vi "SweepStats.vi"(8 "error in (no error)":errorcluster, 10 "Sweep Stats":T1[](array[typedef]), 11 "Action":enum16{"Get", "Set"}(ring)) -> (0 "error out":errorcluster, 2 "sweep stats out":T1[](array[typedef]))   [LabVIEW 2017, in "EmsaWebServiceAccessors.lvlib"]
uses:
  EmsaWebServiceAccessors.lvlib
  SweepStats.ctl
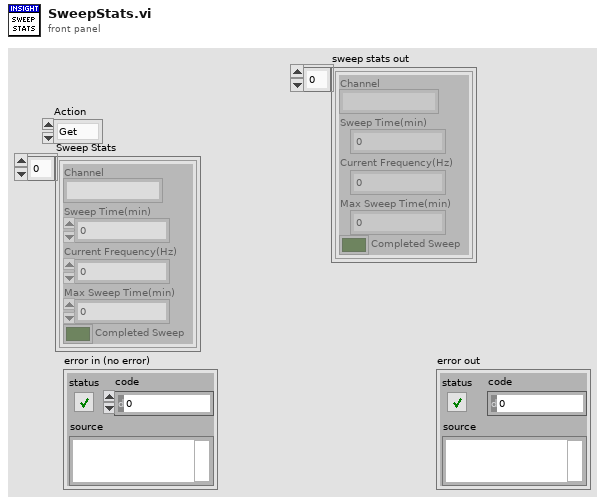
[diagram p1: front panel]
types:
  T1 = typedef "EmsaWebServiceAccessors.lvlib/SweepStats.ctl" = cluster{"Channel":string, "Sweep Time(min)":dbl, "Current Frequency(Hz)":dbl, "Max Sweep Time(min)":dbl, "Completed Sweep":bool}
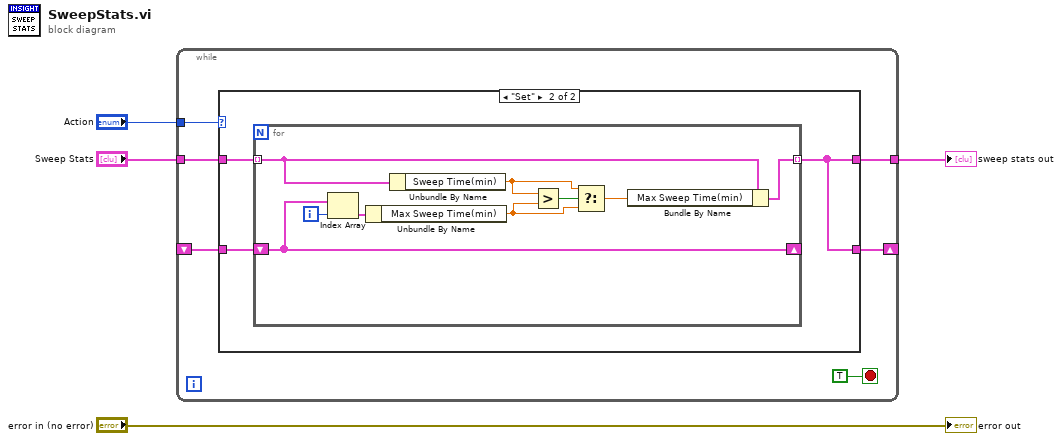
[diagram p0: block diagram]
diagram:
  n1 = while {
    shift-right: [w9] -> _
    shift-left: _ -> [w7]
    tunnel: "Action" -> [w10]
    tunnel: "Sweep Stats" -> [w8]
    tunnel: [w6] -> w2
    stop <- TRUE stop-if-true
    n2 = case shown="\"Set\"" w10 {
      tunnel: [w11 w13] -> w9
      tunnel: w8 -> [_ w14]
      tunnel: w7 -> [w11 w12]
      tunnel: [w11 w13] -> w6
      frame "Get", Default {
      }
      frame "Set" {
        n3 = for {
          tunnel: w14 -> [w16] mode=indexing
          tunnel: [w15] -> w13 mode=indexing
          shift-right: [w21] -> _
          shift-left: w12 -> [w21]
          i -> [w23]
          n4 = Index Array(array=w21, index=w23) -> (element=w22:T1)
          n5 = Unbundle By Name(w22) -> ("Max Sweep Time(min)"=w18:dbl)
          n6 = Unbundle By Name(w16) -> ("Sweep Time(min)"=w19:dbl)
          n7 = Greater?(x=w19, y=w18) -> (0:w20:bool)
          n8 = Select(t=w19, s=w20, f=w18) -> (s? t:f=w17:dbl)
          n9 = Bundle By Name(cluster=w16, "Max Sweep Time(min)"=w17) -> (w15:T1)
        }
      }
    }
  }
  "sweep stats out" <- w2
  "error out" <- "error in (no error)"
